vi "DAQmx Create Channel (TEDS-AI-Strain-Strain Gage).vi"(0 "task in":refnum<k21>, 1 "maximum value":dbl=0.001 format="%0.7f", 2 "minimum value":dbl=-0.001 format="%0.7f", 5 "physical channels":tag, 7 "name to assign":string, 9 "units":i32(ring)=10299 items=["Strain"=10299, "From Custom Scale"=10065], 11 "error in":errorcluster, 12 "custom scale name":tag, 13 "bridge information":T1={"lead wire resistance"=0.0, "initial bridge voltage"=0.0, "voltage excitation source"=10200, "voltage excitation value"=2.5} {"initial bridge voltage" format="%0.2f"; "voltage excitation source" items=["Internal"=10200, "External"=10167, "None"=10230]; "voltage excitation value" format="%0.2f"; "lead wire resistance" format="%0.2f"}) -> (4 "task out":refnum<k21>, 15 "error out":errorcluster)   [LabVIEW 2013]
doc: "Creates channel(s) to measure strain. You must configure the physical channel(s) with TEDS information to use this VI."
uses:
  <resource>/objmgr/daqmx.rc
panel:
  # "input limits"
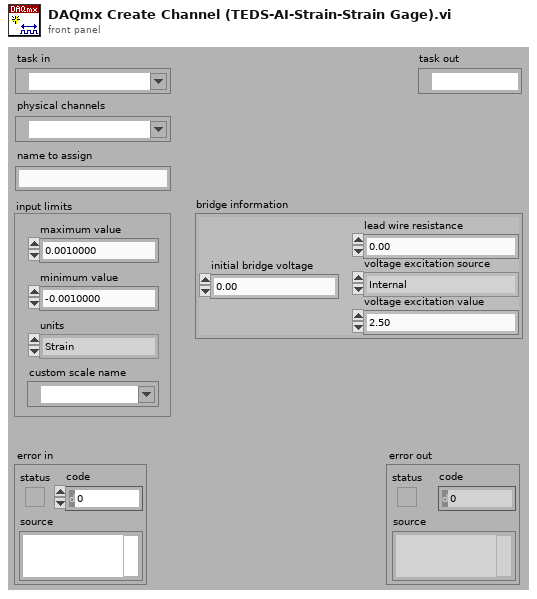
[diagram p1: front panel]
types:
  T1 = cluster{"lead wire resistance":dbl, "initial bridge voltage":dbl, "voltage excitation source":i32, "voltage excitation value":dbl}
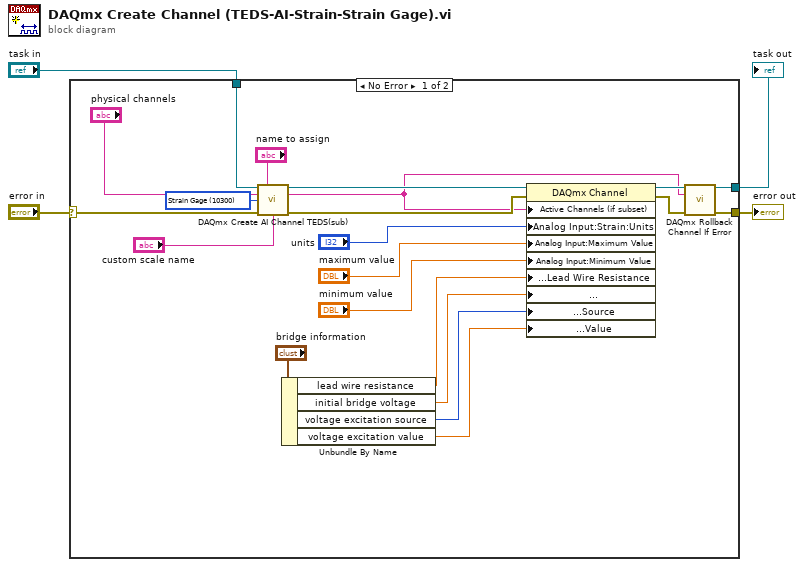
[diagram p0: block diagram]
diagram:
  n1 = case shown="No Error" "error in" {
    selector: "error in" -> [w24 w26]
    tunnel: [w9 w26] -> w4
    tunnel: "task in" -> [w25 w27]
    tunnel: [w8 w27] -> w1
    frame No Error {
      w5 = 10300 items=["Voltage"=10322, "Current"=10134, "More:Voltage:Custom with Excitation"=10323, "More:Current:Custom with Excitation"=10136, "Frequency"=10181, "Period"=10257, "Resistance"=10278, "Temperature:Thermocouple"=10303, "Temperature:Thermistor"=10302, "Temperature:RTD"=10301, "Temperature:Built-in Sensor"=10311, "Strain Gage"=10300, "LVDT"=10352, "RVDT"=10353, "Accelerometer:Voltage Input"=10355, "Accelerometer:Current Input"=10356, "Sound Pressure:Microphone"=10354, "TEDS"=12531] ("measurement type")
      n2 = call "DAQmx Create AI Channel TEDS(sub).vi"("task in"=w25, "virtual channel name"="name to assign", "physical channel name"="physical channels", "measurement type"=w5, "error in"=w24, "custom scale"="custom scale name") -> ("task out"=w22:refnum<k21>, "channel names"=w6:string, "error out"=w17:errorcluster)  [unwired: 7 out]
      n3 = Unbundle By Name("bridge information") -> ("lead wire resistance"=w14:dbl, "initial bridge voltage"=w13:dbl, "voltage excitation source"=w12:i32, "voltage excitation value"=w11:dbl)
      n4 = property class="DAQmx Channel"(reference=w22, error in=w17, "Active Channels (if subset)"=w6, "Analog Input:Strain:Units"="units", "Analog Input:Maximum Value"="maximum value", "Analog Input:Minimum Value"="minimum value", "Analog Input:General Properties:Signal Conditioning:Lead Wire Resistance"=w14, "Analog Input:General Properties:Signal Conditioning:Bridge:Initial Bridge Voltage"=w13, "Analog Input:General Properties:Signal Conditioning:Excitation:Source"=w12, "Analog Input:General Properties:Signal Conditioning:Excitation:Value"=w11) -> (reference out=w10:refnum<k21>, error out=w7:errorcluster)
      n5 = call "DAQmx Rollback Channel If Error.vi"("task in"=w10, "channel names"=w6, "error in"=w7) -> ("task out"=w8:refnum<k21>, "error out"=w9:errorcluster)  [unwired: 11 out]
    }
    frame Error {
    }
  }
  "error out" <- w4
  "task out" <- w1
